vi "Read.vi"(8 "Error In":errorcluster, 10 "UART Channel (0)":u8, 11 "LINX Resource":T2) -> (0 "Error Out":errorcluster, 2 "GPS Data":T1, 3 "LINX Resource":T2)   [LabVIEW 2020, in "LMH-LINX.lvlib" / "PmodGPS.lvlib"]
doc: "Read all data from the PmodGPS. This function returns Time, Date, Status, Fix Type, Satellites in View, Latitude (deg), Longitude (deg), Elevation (m), Ground Speed (km/hr), Ground Speed (knots), and Course over ground (deg)."
uses:
  PmodGPS.lvlib
  Private/Type Defs/LINX Ref.ctl
  Private/Type Defs/Platform.ctl
  Private/Type Defs/Interface.ctl
  Private/Device/Type Defs/LINX Device Config.ctl
  Private/Device/Type Defs/TCP Config.ctl
  Private/Device/Type Defs/Channels.ctl
  Peripherals/UART/UART Read String.vi
  LMH-LINX.lvlib
  Private/Device/Device.lvlib
panel:
  out "Ground Speed (km/hr)":string
  out "Status":string
  out "Ground Speed (knots)":string
  out "Course over ground (degrees)":string
  out "Date":string
  out "Satellites in View":string
  out "Fix Type":string
  in  "Time Fix (Add)":i32=-7
  out "Longitude (deg)":string
  out "Latitude (deg)":string
  out "Time":string
  out "Elevation (m)":string
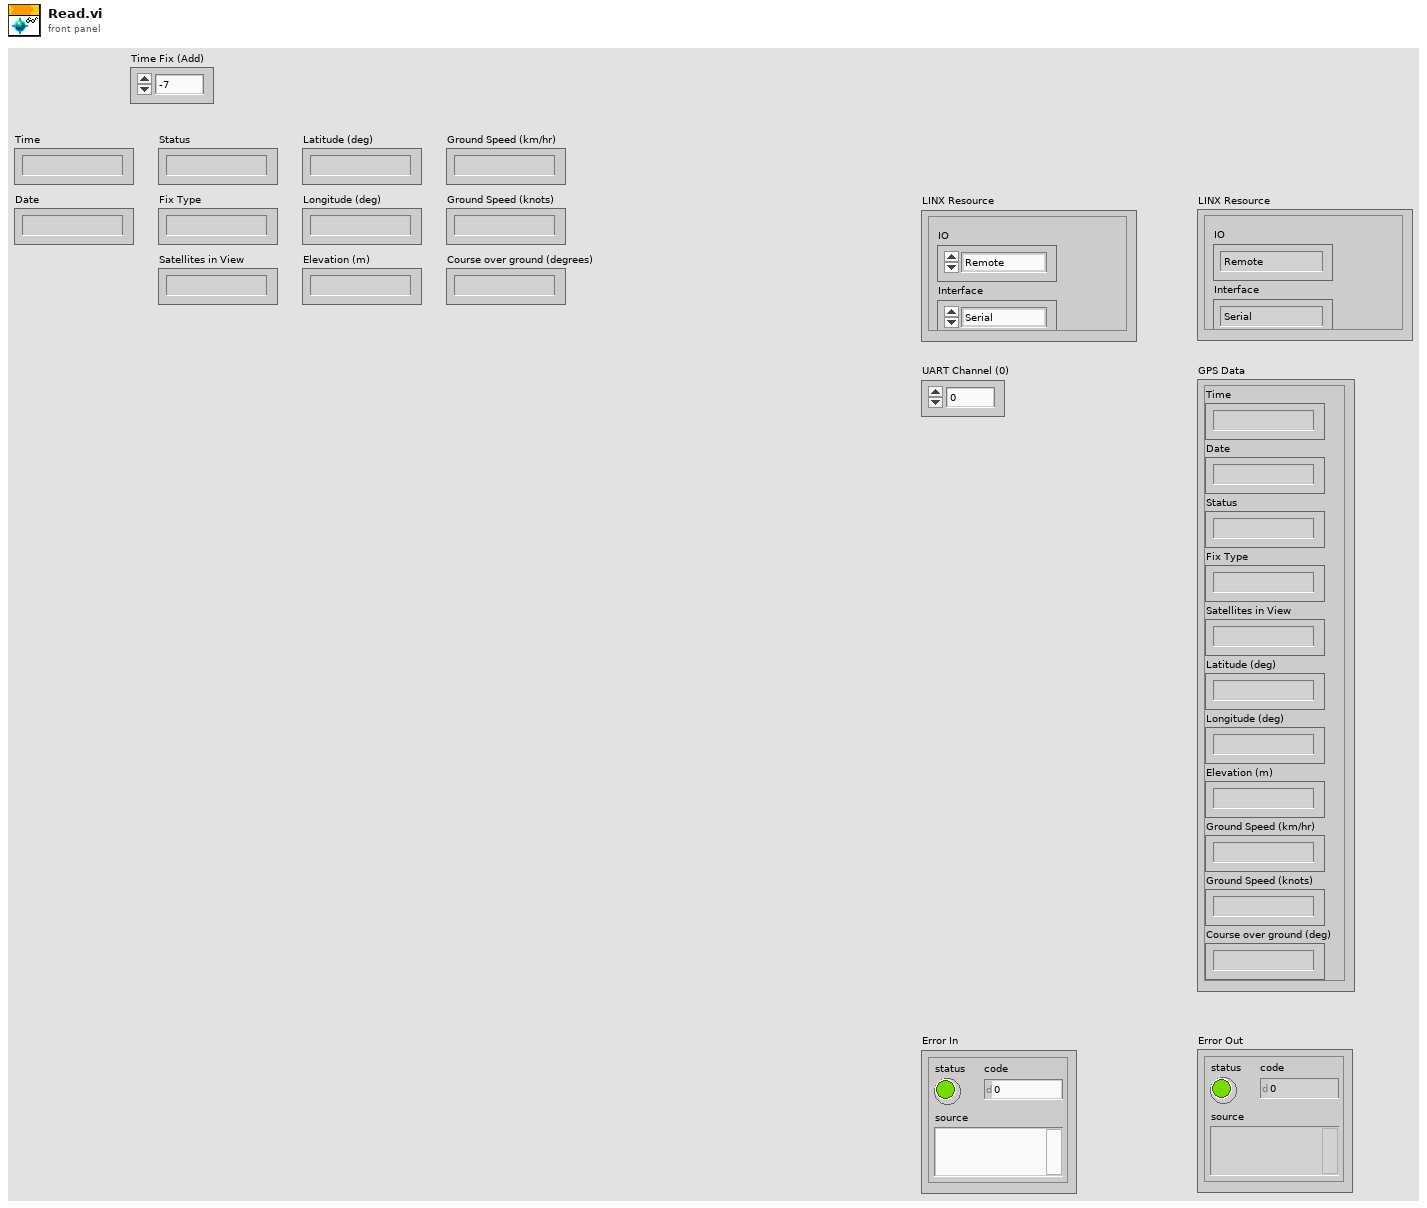
[diagram p1: front panel]
types:
  T1 = cluster{"Time":string, "Date":string, "Status":string, "Fix Type":string, "Satellites in View":string, "Latitude (deg)":string, "Longitude (deg)":string, "Elevation (m)":string, "Ground Speed (km/hr)":string, "Ground Speed (knots)":string, "Course over ground (deg)":string}
  T2 = typedef "LMH-LINX.lvlib/LINX Ref.ctl" = cluster{"IO":T3, "Interface":T4, "LINX Device Config":T5}
  T3 = typedef "LMH-LINX.lvlib/Platform.ctl" = enum16{"Remote", "Local"}
  T4 = typedef "LMH-LINX.lvlib/Interface.ctl" = enum16{"Serial", "TCP"}
  T5 = typedef "LMH-LINX.lvlib/Device.lvlib/LINX Device Config.ctl" = cluster{"Interface":T4, "COM Port":refnum<visa-resource-name>, "TCP Configuration":T6, "Device Family":u8, "Device ID":u8, "Device Name":string, "TCP Ref":refnum<k5>, "Channels":T7}
  T6 = typedef "LMH-LINX.lvlib/Device.lvlib/TCP Config.ctl" = cluster{"IP Address":string, "Port":u16}
  T7 = typedef "LMH-LINX.lvlib/Channels.ctl" = cluster{"DI":u8[], "DO":u8[], "AI":u8[], "AO":u8[], "PWM":u8[], "QE":u8[], "UART":u8[], "I2C 2":u8[], "SPI":u8[], "CAN":u8[], "Servo":u8[], "AI Ref (V)":dbl, "AI Resolution (Bits)":u8, "AO Ref (V)":dbl, "AO Resolution (Bits)":u8}
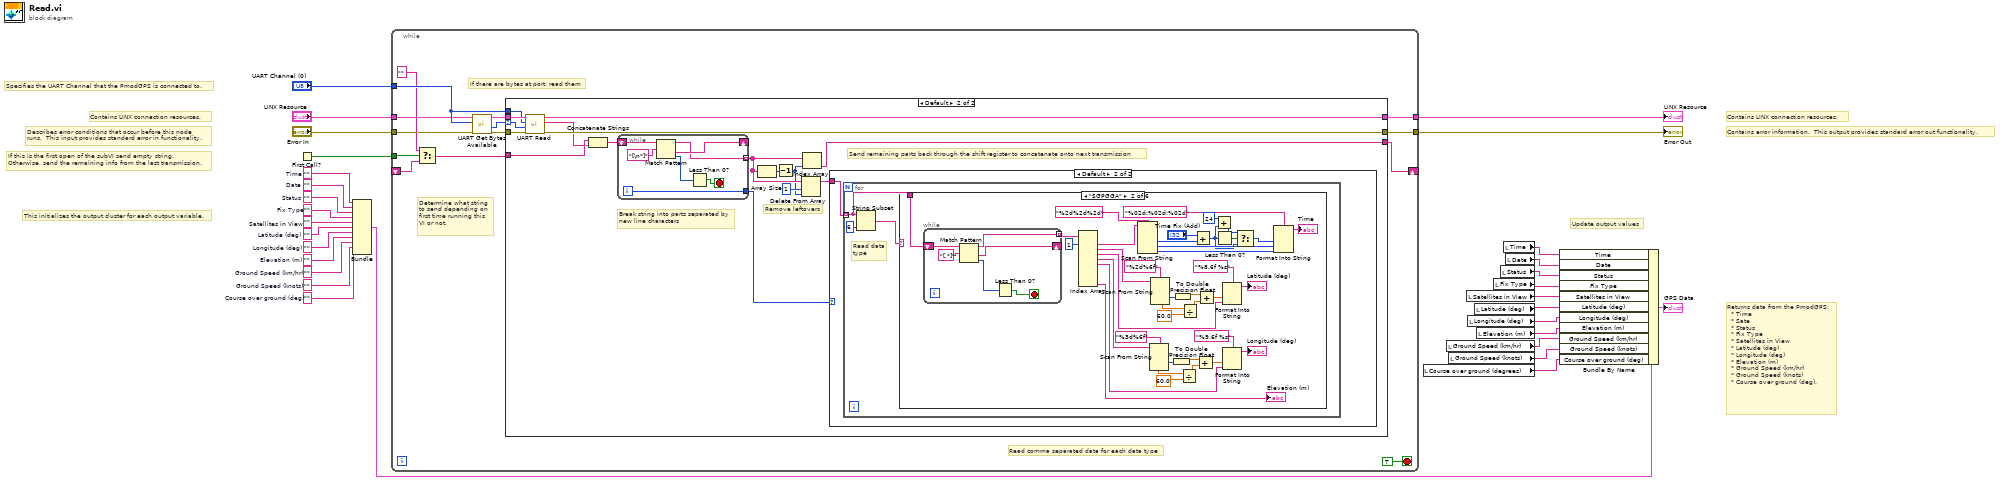
[diagram p0: block diagram]
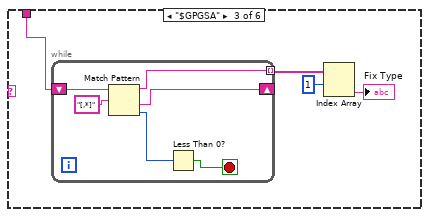
[diagram p5: hidden frame]
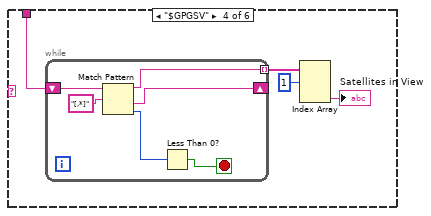
[diagram p6: hidden frame]
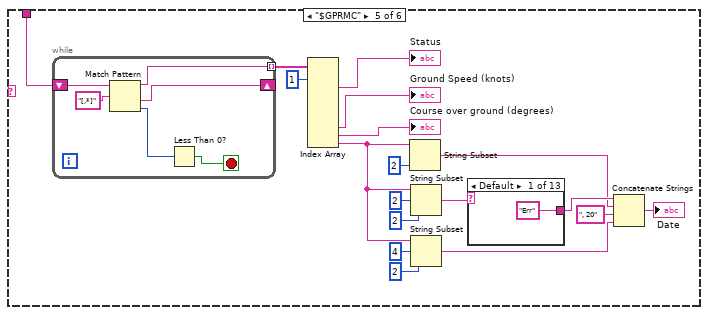
[diagram p7: hidden frame]
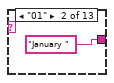
[diagram p8: hidden frame]
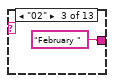
[diagram p9: hidden frame]
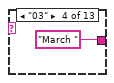
[diagram p10: hidden frame]
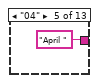
[diagram p11: hidden frame]
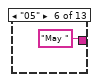
[diagram p12: hidden frame]
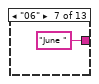
[diagram p13: hidden frame]
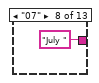
[diagram p14: hidden frame]
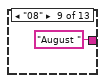
[diagram p15: hidden frame]
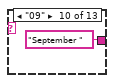
[diagram p16: hidden frame]
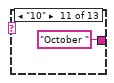
[diagram p17: hidden frame]
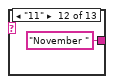
[diagram p18: hidden frame]
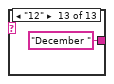
[diagram p19: hidden frame]
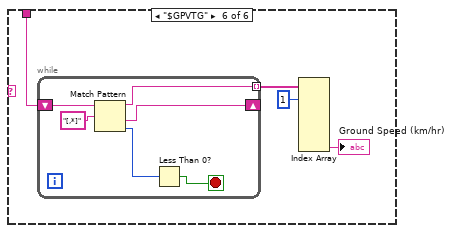
[diagram p20: hidden frame]
diagram:
  w14 = ""  # Course over ground (deg)
  w15 = ""  # Ground Speed (knots)
  w16 = ""  # Ground Speed (km/hr)
  w17 = ""  # Elevation (m)
  w18 = ""  # Longitude (deg)
  w19 = ""  # Latitude (deg)
  w20 = ""  # Satellites in View
  w21 = ""  # Fix Type
  w22 = ""  # Status
  w23 = ""  # Date
  w24 = ""  # Time
  # "If this is the first open of the subVI send empty string.\nOtherwise, send the remaining info from the last transmission."
  # "Update output values"
  # "Returns data from the PmodGPS:\n  * Time\n  * Sate\n  * Status\n  * Fix Type\n  * Satellites in View\n  * Latitude (deg)\n  * Longitude (deg)\n  * Elevation (m)\n  * Ground Speed (km/hr)\n  * Ground Speed (knots)\n  * Course over ground (deg)."
  # "Contains error information.  This output provides standard error out functionality."
  # "Contains LINX connection resources."
  # "This initializes the output cluster for each output variable."
  # "Describes error conditions that occur before this node\nruns.  This input provides standard error in functionality."
  # "Contains LINX connection resources."
  # "Specifies the UART Channel that the PmodGPS is connected to."
  n1 = First Call?() -> (First Call?: T/F=w29:bool)
  n2 = Bundle("Time"=w24, "Date"=w23, "Status"=w22, "Fix Type"=w21, "Satellites in View"=w20, "Latitude (deg)"=w19, "Longitude (deg)"=w18, "Elevation (m)"=w17, "Ground Speed (km/hr)"=w16, "Ground Speed (knots)"=w15, "Course over ground (deg)"=w14) -> (w13:T1)  [unwired: 1 in]
  n3 = while {
    shift-right: [w40] -> _
    shift-left: _ -> [w36]
    tunnel: "UART Channel (0)" -> [w39]
    tunnel: w29 -> [w38]
    tunnel: "LINX Resource" -> [w34]
    tunnel: "Error In" -> [w33]
    tunnel: [w32] -> w26
    tunnel: [w31] -> w25
    stop <- TRUE stop-if-true
    # "Read comma separated data for each data type"
    # "If there are bytes at port, read them"
    # "Determine what string\nto send depending on \nfirst time running this\nVI or not."
    n4 = Select(t="", s=w38, f=w36) -> (s? t:f=w35:string)
    n5 = call "UART Get Bytes Available.vi"("Error In"=w33, "UART Channel (0)"=w39, "LINX Resource"=w34) -> ("Error Out"=w44:errorcluster, "Bytes Available"=w42:u8, "LINX Resource"=w43:T2)  [unwired: 6 in]
    n6 = case shown="Default" w42 {
      selector: w42 -> [_ w59]
      tunnel: w44 -> [w46 w63]
      tunnel: w43 -> [w47 w62]
      tunnel: [w47 w61] -> w32
      tunnel: [w46 w60] -> w31
      tunnel: [w45 w50] -> w40
      tunnel: w35 -> [w45 w58]
      tunnel: w39 -> [_ w49]
      frame 0 {
      }
      frame Default {
        # "Remove leftovers"
        # "Send remaining parts back through the shift register to concatenate onto next transmission"
        # "Break string into parts separated by\nnew line characters"
        n7 = call-poly "UART Read.vi"("Error In"=w63, "Num Bytes"=w59, "UART Channel (0)"=w49, "LINX Resource"=w62) -> ("Error Out"=w60:errorcluster, "Data"=w48:string, "LINX Resource"=w61:T2)  [unwired: 5 in]
        n8 = Concatenate Strings(w58, w48) -> (w57:string)
        n9 = while {
          shift-right: [w182] -> _
          shift-left: w57 -> [w186]
          tunnel: [w181] -> w55 mode=indexing
          tunnel: [w180] -> w56
          i -> [w180]
          stop <- w184 stop-if-true
          n10 = Match Pattern(string=w186, regular expression="[\n*]") -> (before substring=w181:string, after substring=w182:string, offset past match=w183:i32)  [unwired: 1 in, 1 out]
          n11 = Less Than 0?(x=w183) -> (x < 0?=w184:bool)
        }
        n12 = Array Size(array=w55) -> (size(s)=w53:i32)
        n13 = Decrement(x=w53) -> (x-1=w52:i32)
        n14 = Delete From Array(array=w55, length=1, index=w52) -> (array with subset deleted=w51:string[])  [unwired: 1 out]
        n15 = Index Array(array=w55, index=w52) -> (element=w50:string)
        n16 = case shown="Default" w56 {
          tunnel: w51 -> [_ w64]
          frame 0 {
          }
          frame Default {
            n17 = for {
              tunnel: w64 -> [w65] mode=indexing
              # "Read data\ntype"
              n18 = String Subset(string=w65, length (rest)=6 ("length (rest)")) -> (substring=w66:string)  [unwired: 1 in]
              n19 = case shown="\"$GPGGA\"" w66 {
                tunnel: w65 -> [_ w106 w116 w126 w150 w173]
                frame Default {
                }
                frame "$GPGGA" {
                  n20 = while {
                    shift-right: [w108] -> _
                    shift-left: w106 -> [w110]
                    tunnel: [w107] -> w105 mode=indexing
                    stop <- w112 stop-if-true
                    n21 = Match Pattern(string=w110, regular expression="[,*]") -> (before substring=w107:string, after substring=w108:string, offset past match=w111:i32)  [unwired: 1 in, 1 out]
                    n22 = Less Than 0?(x=w111) -> (x < 0?=w112:bool)
                  }
                  n23 = Index Array(array=w105, index #1=1 ("index")) -> (element #1=w103:string, element #2=w96:string, element #3=w88:string, element #4=w87:string, element #5=w86:string, element #9=→"Elevation (m)":string)  [unwired: 8 in, 3 out]
                  n24 = Scan From String(format string="%2d%2d%2d", input string=w103) -> (output 1=w102:i32, output 2=w100:i32, output 3=w99:i32)  [unwired: 5 in, 3 out]
                  n25 = Scan From String(format string="%3d%6f", input string=w87) -> (output 1=w83:i32, output 2=w84:dbl)  [unwired: 4 in, 3 out]
                  n26 = Scan From String(format string="%2d%6f", input string=w96) -> (output 1=w94:i32, output 2=w91:dbl)  [unwired: 4 in, 3 out]
                  n27 = To Double Precision Float(number=w83) -> (double precision float=w82:dbl)
                  n28 = To Double Precision Float(number=w94) -> (double precision float=w93:dbl)
                  n29 = Divide(x=w84, y=60.0) -> (x/y=w81:dbl)
                  n30 = Divide(x=w91, y=60.0) -> (x/y=w90:dbl)
                  n31 = Add(x="Time Fix (Add)", y=w102) -> (x+y=w69:i32)
                  n32 = Add(x=w82, y=w81) -> (x+y=w79:dbl)
                  n33 = Add(x=w93, y=w90) -> (x+y=w89:dbl)
                  n34 = Add(x=24, y=w69) -> (x+y=w71:i32)
                  n35 = Less Than 0?(x=w69) -> (x < 0?=w73:bool)
                  n36 = Format Into String(format string="%8.6f %s", w89, w88) -> (resulting string=→"Latitude (deg)":string)  [unwired: 2 in, 1 out]
                  n37 = Format Into String(format string="%9.6f %s", w79, w86) -> (resulting string=→"Longitude (deg)":string)  [unwired: 2 in, 1 out]
                  n38 = Select(t=w71, s=w73, f=w69) -> (s? t:f=w70:i32)
                  n39 = Format Into String(format string="%02d:%02d:%02d", w70, w100, w99) -> (resulting string=→"Time":string)  [unwired: 2 in, 1 out]
                }
                frame "$GPGSA" {
                  n40 = while {
                    shift-right: [w118] -> _
                    shift-left: w116 -> [w120]
                    tunnel: [w117] -> w115 mode=indexing
                    stop <- w122 stop-if-true
                    n41 = Match Pattern(string=w120, regular expression="[,*]") -> (before substring=w117:string, after substring=w118:string, offset past match=w121:i32)  [unwired: 1 in, 1 out]
                    n42 = Less Than 0?(x=w121) -> (x < 0?=w122:bool)
                  }
                  n43 = Index Array(array=w115, index #1=1 ("index")) -> (element #2=→"Fix Type":string)  [unwired: 1 in, 1 out]
                }
                frame "$GPGSV" {
                  n44 = while {
                    shift-right: [w128] -> _
                    shift-left: w126 -> [w130]
                    tunnel: [w127] -> w125 mode=indexing
                    stop <- w132 stop-if-true
                    n45 = Match Pattern(string=w130, regular expression="[,*]") -> (before substring=w127:string, after substring=w128:string, offset past match=w131:i32)  [unwired: 1 in, 1 out]
                    n46 = Less Than 0?(x=w131) -> (x < 0?=w132:bool)
                  }
                  n47 = Index Array(array=w125, index #1=1 ("index")) -> (element #3=→"Satellites in View":string)  [unwired: 2 in, 2 out]
                }
                frame "$GPRMC" {
                  n48 = while {
                    shift-right: [w165] -> _
                    shift-left: w150 -> [w167]
                    tunnel: [w164] -> w149 mode=indexing
                    stop <- w169 stop-if-true
                    n49 = Match Pattern(string=w167, regular expression="[,*]") -> (before substring=w164:string, after substring=w165:string, offset past match=w168:i32)  [unwired: 1 in, 1 out]
                    n50 = Less Than 0?(x=w168) -> (x < 0?=w169:bool)
                  }
                  n51 = Index Array(array=w149, index #1=1 ("index")) -> (element #2=→"Status":string, element #7=→"Ground Speed (knots)":string, element #8=→"Course over ground (degrees)":string, element #9=w144:string)  [unwired: 8 in, 5 out]
                  n52 = String Subset(string=w144, length (rest)=2 ("length (rest)")) -> (substring=w136:string)  [unwired: 1 in]
                  n53 = String Subset(string=w144, offset (0)=2, length (rest)=2 ("length (rest)")) -> (substring=w138:string)
                  n54 = String Subset(string=w144, offset (0)=4, length (rest)=2 ("length (rest)")) -> (substring=w134:string)
                  n55 = case shown="Default" w138 {
                    tunnel: ["Err" "January " "February " "March " "April " "May " "June " "July " "August " "September " "October " "November " "December "] -> w137
                    frame Default {
                    }
                    frame "01" {
                    }
                    frame "02" {
                    }
                    frame "03" {
                    }
                    frame "04" {
                    }
                    frame "05" {
                    }
                    frame "06" {
                    }
                    frame "07" {
                    }
                    frame "08" {
                    }
                    frame "09" {
                    }
                    frame "10" {
                    }
                    frame "11" {
                    }
                    frame "12" {
                    }
                  }
                  n56 = Concatenate Strings(w137, w136, ", 20" ("string"), w134) -> (→"Date":string)
                }
                frame "$GPVTG" {
                  n57 = while {
                    shift-right: [w175] -> _
                    shift-left: w173 -> [w177]
                    tunnel: [w174] -> w172 mode=indexing
                    stop <- w179 stop-if-true
                    n58 = Match Pattern(string=w177, regular expression="[,*]") -> (before substring=w174:string, after substring=w175:string, offset past match=w178:i32)  [unwired: 1 in, 1 out]
                    n59 = Less Than 0?(x=w178) -> (x < 0?=w179:bool)
                  }
                  n60 = Index Array(array=w172, index #1=1 ("index")) -> (element #7=→"Ground Speed (km/hr)":string)  [unwired: 6 in, 6 out]
                }
              }
            }
          }
        }
      }
    }
  }
  "LINX Resource" <- w26
  "Error Out" <- w25
  n61 = local read "Course over ground (degrees)"() -> (w2:string)
  n62 = local read "Ground Speed (km/hr)"() -> (w4:string)
  n63 = local read "Ground Speed (knots)"() -> (w3:string)
  n64 = local read "Satellites in View"() -> (w8:string)
  n65 = local read "Longitude (deg)"() -> (w6:string)
  n66 = local read "Latitude (deg)"() -> (w7:string)
  n67 = local read "Elevation (m)"() -> (w5:string)
  n68 = local read "Fix Type"() -> (w9:string)
  n69 = local read "Status"() -> (w10:string)
  n70 = local read "Time"() -> (w12:string)
  n71 = local read "Date"() -> (w11:string)
  n72 = Bundle By Name(cluster=w13, "Time"=w12, "Date"=w11, "Status"=w10, "Fix Type"=w9, "Satellites in View"=w8, "Latitude (deg)"=w7, "Longitude (deg)"=w6, "Elevation (m)"=w5, "Ground Speed (km/hr)"=w4, "Ground Speed (knots)"=w3, "Course over ground (deg)"=w2) -> (→"GPS Data":T1)
